vi "normal (SubVI).vi"(6 "seed":i32=-1, 7 "reset":bool=TRUE, 9 "std":dbl=1.0, 10 "mean":dbl) -> ()   [LabVIEW 2011]
panel:
  out "Array":cluster{"x":dbl, "y":dbl}[](array[cluster])
  in  "samples":i32=-1
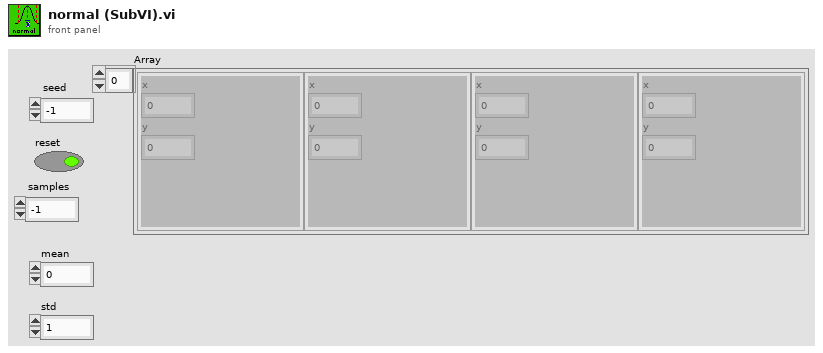
[diagram p1: front panel]
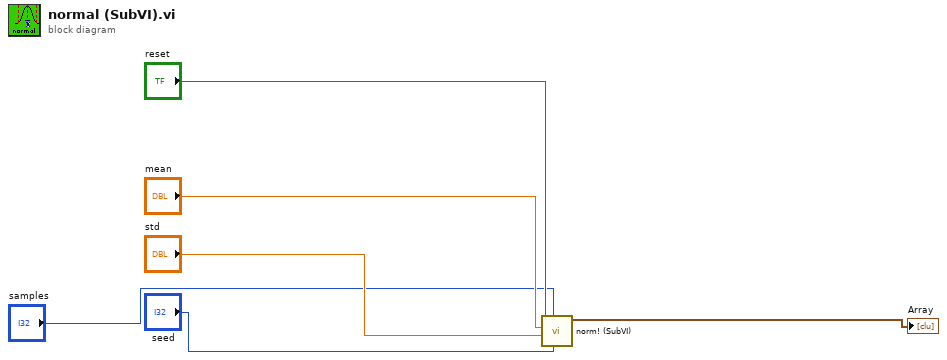
[diagram p0: block diagram]
diagram:
  n1 = call "norm! (SubVI).vi"("seed"="seed", "samples"="samples", "std"="std", "mean"="mean", "reset"="reset") -> ("Array"=→"Array":cluster{"x":dbl, "y":dbl}[])  [unwired: 6 in]
